vi "Lab Panel V4.82.vi"() -> ()   [LabVIEW 2013] (continued)
                n968 = Less?(x=w1637, y=2) -> (x < y?=w1640:bool)
                n969 = local read "DISP LAB02-2"() -> (w1642:T4)
                n970 = Unbundle(w1642) -> ("STATUS"=w1643:string)  [unwired: 2 out]
                n971 = Equal?(x=w1643, y="RUN") -> (x = y?=w1639:bool)
                n972 = And(x=w1639, y=w1640) -> (x .and. y?=w1638:bool)
                n973 = case shown="True" w1638 {
                  tunnel: w1642 -> [_ w1648]
                  tunnel: w1637 -> [_ w1652]
                  frame False {
                  }
                  frame True {
                    n974 = local read "SET LAB02-2"() -> (w1654:T5)
                    n975 = local read "TDMS LAB02-2"() -> (w1647:refnum<k34>)
                    n976 = Unbundle(w1648) -> ("CYCLE"=w1653:dbl)  [unwired: 2 out]
                    n977 = Unbundle(w1654) -> ("CYCLES"=w1645:dbl, "T-RISE mins"=w1651:dbl)  [unwired: 3 out]
                    n978 = case shown="\"T-RISE TEST\"" w1652 {
                      tunnel: w1651 -> [_ _ w1661]
                      tunnel: [w1656 w1658 w1661] -> w1650
                      tunnel: w1645 -> [w1656 w1658 _]
                      tunnel: ["CHART PASS" "CYCLE PASS" "T-RISE PASS"] -> w1649
                      frame "CHART TEST", Default {
                      }
                      frame "CYCLE TEST" {
                      }
                      frame "T-RISE TEST" {
                      }
                    }
                    n979 = Increment(x=w1645) -> (x+1=w1646:dbl)
                    n980 = Greater Or Equal?(x=w1653, y=w1646) -> (x >= y?=w1655:bool)
                    n981 = case shown="True" w1655 {
                      tunnel: w1650 -> [w1665 _]
                      tunnel: w1649 -> [w1664 _]
                      tunnel: w1648 -> [w1663 _]
                      tunnel: w1647 -> [w1662 _]
                      frame True {
                        n982 = stacked-sequence {
                          tunnel: w1665 -> [w1669 _]
                          tunnel: w1664 -> [w1667 w1673]
                          tunnel: w1663 -> [_ w1676]
                          tunnel: w1662 -> [w1666 _]
                          frame #0 {
                            n983 = Build Array(w1667) -> (w1670:string[])
                            n984 = Build Array(w1669) -> (w1668:dbl[])
                            n985 = TDMS Write(0:w1666, 5:"TEST PASS", 7:w1670, 9:w1668) -> (15:w1672:errorcluster)  [unwired: 2 in, 3 out]
                            n986 = local write "data file error"(w1672) -> ()
                          }
                          frame #1 {
                            n987 = Bundle(cluster=w1676, "STATUS"=w1673) -> (w1674:T4)  [unwired: 2 in]
                            n988 = local write "RESULT LAB02-2"(TRUE) -> ()
                            n989 = local write "DISP LAB02-2"(w1674) -> ()
                          }
                        }
                      }
                      frame False {
                      }
                    }
                  }
                }
              }
              frame #4 {
                # "LAB03-1"
                n990 = Less?(x=w1677, y=2) -> (x < y?=w1680:bool)
                n991 = local read "DISP LAB03-1"() -> (w1682:T4)
                n992 = Unbundle(w1682) -> ("STATUS"=w1683:string)  [unwired: 2 out]
                n993 = Equal?(x=w1683, y="RUN") -> (x = y?=w1679:bool)
                n994 = And(x=w1679, y=w1680) -> (x .and. y?=w1678:bool)
                n995 = case shown="True" w1678 {
                  tunnel: w1682 -> [_ w1688]
                  tunnel: w1677 -> [_ w1692]
                  frame False {
                  }
                  frame True {
                    n996 = local read "SET LAB03-1"() -> (w1694:T5)
                    n997 = local read "TDMS LAB03-1"() -> (w1687:refnum<k34>)
                    n998 = Unbundle(w1688) -> ("CYCLE"=w1693:dbl)  [unwired: 2 out]
                    n999 = Unbundle(w1694) -> ("CYCLES"=w1685:dbl, "T-RISE mins"=w1691:dbl)  [unwired: 3 out]
                    n1000 = case shown="\"T-RISE TEST\"" w1692 {
                      tunnel: w1691 -> [_ _ w1701]
                      tunnel: [w1696 w1698 w1701] -> w1690
                      tunnel: w1685 -> [w1696 w1698 _]
                      tunnel: ["CHART PASS" "CYCLE PASS" "T-RISE PASS"] -> w1689
                      frame "CHART TEST", Default {
                      }
                      frame "CYCLE TEST" {
                      }
                      frame "T-RISE TEST" {
                      }
                    }
                    n1001 = Increment(x=w1685) -> (x+1=w1686:dbl)
                    n1002 = Greater Or Equal?(x=w1693, y=w1686) -> (x >= y?=w1695:bool)
                    n1003 = case shown="True" w1695 {
                      tunnel: w1690 -> [w1705 _]
                      tunnel: w1689 -> [w1704 _]
                      tunnel: w1688 -> [w1703 _]
                      tunnel: w1687 -> [w1702 _]
                      frame True {
                        n1004 = stacked-sequence {
                          tunnel: w1705 -> [w1709 _]
                          tunnel: w1704 -> [w1707 w1713]
                          tunnel: w1703 -> [_ w1716]
                          tunnel: w1702 -> [w1706 _]
                          frame #0 {
                            n1005 = Build Array(w1707) -> (w1710:string[])
                            n1006 = Build Array(w1709) -> (w1708:dbl[])
                            n1007 = TDMS Write(0:w1706, 5:"TEST PASS", 7:w1710, 9:w1708) -> (15:w1712:errorcluster)  [unwired: 2 in, 3 out]
                            n1008 = local write "data file error"(w1712) -> ()
                          }
                          frame #1 {
                            n1009 = Bundle(cluster=w1716, "STATUS"=w1713) -> (w1714:T4)  [unwired: 2 in]
                            n1010 = local write "RESULT LAB03-1"(TRUE) -> ()
                            n1011 = local write "DISP LAB03-1"(w1714) -> ()
                          }
                        }
                      }
                      frame False {
                      }
                    }
                  }
                }
              }
              frame #5 {
                # "LAB03-2"
                n1012 = Less?(x=w1717, y=2) -> (x < y?=w1720:bool)
                n1013 = local read "DISP LAB03-2"() -> (w1722:T4)
                n1014 = Unbundle(w1722) -> ("STATUS"=w1723:string)  [unwired: 2 out]
                n1015 = Equal?(x=w1723, y="RUN") -> (x = y?=w1719:bool)
                n1016 = And(x=w1719, y=w1720) -> (x .and. y?=w1718:bool)
                n1017 = case shown="True" w1718 {
                  tunnel: w1722 -> [_ w1728]
                  tunnel: w1717 -> [_ w1732]
                  frame False {
                  }
                  frame True {
                    n1018 = local read "SET LAB03-2"() -> (w1734:T5)
                    n1019 = local read "TDMS LAB03-2"() -> (w1727:refnum<k34>)
                    n1020 = Unbundle(w1728) -> ("CYCLE"=w1733:dbl)  [unwired: 2 out]
                    n1021 = Unbundle(w1734) -> ("CYCLES"=w1725:dbl, "T-RISE mins"=w1731:dbl)  [unwired: 3 out]
                    n1022 = case shown="\"T-RISE TEST\"" w1732 {
                      tunnel: w1731 -> [_ _ w1741]
                      tunnel: [w1736 w1738 w1741] -> w1730
                      tunnel: w1725 -> [w1736 w1738 _]
                      tunnel: ["CHART PASS" "CYCLE PASS" "T-RISE PASS"] -> w1729
                      frame "CHART TEST", Default {
                      }
                      frame "CYCLE TEST" {
                      }
                      frame "T-RISE TEST" {
                      }
                    }
                    n1023 = Increment(x=w1725) -> (x+1=w1726:dbl)
                    n1024 = Greater Or Equal?(x=w1733, y=w1726) -> (x >= y?=w1735:bool)
                    n1025 = case shown="True" w1735 {
                      tunnel: w1730 -> [w1745 _]
                      tunnel: w1729 -> [w1744 _]
                      tunnel: w1728 -> [w1743 _]
                      tunnel: w1727 -> [w1742 _]
                      frame True {
                        n1026 = stacked-sequence {
                          tunnel: w1745 -> [w1749 _]
                          tunnel: w1744 -> [w1747 w1753]
                          tunnel: w1743 -> [_ w1756]
                          tunnel: w1742 -> [w1746 _]
                          frame #0 {
                            n1027 = Build Array(w1747) -> (w1750:string[])
                            n1028 = Build Array(w1749) -> (w1748:dbl[])
                            n1029 = TDMS Write(0:w1746, 5:"TEST PASS", 7:w1750, 9:w1748) -> (15:w1752:errorcluster)  [unwired: 2 in, 3 out]
                            n1030 = local write "data file error"(w1752) -> ()
                          }
                          frame #1 {
                            n1031 = Bundle(cluster=w1756, "STATUS"=w1753) -> (w1754:T4)  [unwired: 2 in]
                            n1032 = local write "RESULT LAB03-2"(TRUE) -> ()
                            n1033 = local write "DISP LAB03-2"(w1754) -> ()
                          }
                        }
                      }
                      frame False {
                      }
                    }
                  }
                }
              }
              frame #6 {
                # "LAB04-1"
                n1034 = Less?(x=w1757, y=2) -> (x < y?=w1760:bool)
                n1035 = local read "DISP LAB04-1"() -> (w1762:T4)
                n1036 = Unbundle(w1762) -> ("STATUS"=w1763:string)  [unwired: 2 out]
                n1037 = Equal?(x=w1763, y="RUN") -> (x = y?=w1759:bool)
                n1038 = And(x=w1759, y=w1760) -> (x .and. y?=w1758:bool)
                n1039 = case shown="True" w1758 {
                  tunnel: w1762 -> [_ w1768]
                  tunnel: w1757 -> [_ w1772]
                  frame False {
                  }
                  frame True {
                    n1040 = local read "SET LAB04-1"() -> (w1774:T5)
                    n1041 = local read "TDMS LAB04-1"() -> (w1767:refnum<k34>)
                    n1042 = Unbundle(w1768) -> ("CYCLE"=w1773:dbl)  [unwired: 2 out]
                    n1043 = Unbundle(w1774) -> ("CYCLES"=w1765:dbl, "T-RISE mins"=w1771:dbl)  [unwired: 3 out]
                    n1044 = case shown="\"T-RISE TEST\"" w1772 {
                      tunnel: w1771 -> [_ _ w1781]
                      tunnel: [w1776 w1778 w1781] -> w1770
                      tunnel: w1765 -> [w1776 w1778 _]
                      tunnel: ["CHART PASS" "CYCLE PASS" "T-RISE PASS"] -> w1769
                      frame "CHART TEST", Default {
                      }
                      frame "CYCLE TEST" {
                      }
                      frame "T-RISE TEST" {
                      }
                    }
                    n1045 = Increment(x=w1765) -> (x+1=w1766:dbl)
                    n1046 = Greater Or Equal?(x=w1773, y=w1766) -> (x >= y?=w1775:bool)
                    n1047 = case shown="True" w1775 {
                      tunnel: w1770 -> [w1785 _]
                      tunnel: w1769 -> [w1784 _]
                      tunnel: w1768 -> [w1783 _]
                      tunnel: w1767 -> [w1782 _]
                      frame True {
                        n1048 = stacked-sequence {
                          tunnel: w1785 -> [w1789 _]
                          tunnel: w1784 -> [w1787 w1793]
                          tunnel: w1783 -> [_ w1796]
                          tunnel: w1782 -> [w1786 _]
                          frame #0 {
                            n1049 = Build Array(w1787) -> (w1790:string[])
                            n1050 = Build Array(w1789) -> (w1788:dbl[])
                            n1051 = TDMS Write(0:w1786, 5:"TEST PASS", 7:w1790, 9:w1788) -> (15:w1792:errorcluster)  [unwired: 2 in, 3 out]
                            n1052 = local write "data file error"(w1792) -> ()
                          }
                          frame #1 {
                            n1053 = Bundle(cluster=w1796, "STATUS"=w1793) -> (w1794:T4)  [unwired: 2 in]
                            n1054 = local write "RESULT LAB04-1"(TRUE) -> ()
                            n1055 = local write "DISP LAB04-1"(w1794) -> ()
                          }
                        }
                      }
                      frame False {
                      }
                    }
                  }
                }
              }
              frame #7 {
                # "LAB04-2"
                n1056 = Less?(x=w1797, y=2) -> (x < y?=w1800:bool)
                n1057 = local read "DISP LAB04-2"() -> (w1802:T4)
                n1058 = Unbundle(w1802) -> ("STATUS"=w1803:string)  [unwired: 2 out]
                n1059 = Equal?(x=w1803, y="RUN") -> (x = y?=w1799:bool)
                n1060 = And(x=w1799, y=w1800) -> (x .and. y?=w1798:bool)
                n1061 = case shown="True" w1798 {
                  tunnel: w1802 -> [_ w1808]
                  tunnel: w1797 -> [_ w1812]
                  frame False {
                  }
                  frame True {
                    n1062 = local read "SET LAB04-2"() -> (w1814:T5)
                    n1063 = local read "TDMS LAB04-2"() -> (w1807:refnum<k34>)
                    n1064 = Unbundle(w1808) -> ("CYCLE"=w1813:dbl)  [unwired: 2 out]
                    n1065 = Unbundle(w1814) -> ("CYCLES"=w1805:dbl, "T-RISE mins"=w1811:dbl)  [unwired: 3 out]
                    n1066 = case shown="\"T-RISE TEST\"" w1812 {
                      tunnel: w1811 -> [_ _ w1821]
                      tunnel: [w1816 w1818 w1821] -> w1810
                      tunnel: w1805 -> [w1816 w1818 _]
                      tunnel: ["CHART PASS" "CYCLE PASS" "T-RISE PASS"] -> w1809
                      frame "CHART TEST", Default {
                      }
                      frame "CYCLE TEST" {
                      }
                      frame "T-RISE TEST" {
                      }
                    }
                    n1067 = Increment(x=w1805) -> (x+1=w1806:dbl)
                    n1068 = Greater Or Equal?(x=w1813, y=w1806) -> (x >= y?=w1815:bool)
                    n1069 = case shown="True" w1815 {
                      tunnel: w1810 -> [w1825 _]
                      tunnel: w1809 -> [w1824 _]
                      tunnel: w1808 -> [w1823 _]
                      tunnel: w1807 -> [w1822 _]
                      frame True {
                        n1070 = stacked-sequence {
                          tunnel: w1825 -> [w1829 _]
                          tunnel: w1824 -> [w1827 w1833]
                          tunnel: w1823 -> [_ w1836]
                          tunnel: w1822 -> [w1826 _]
                          frame #0 {
                            n1071 = Build Array(w1827) -> (w1830:string[])
                            n1072 = Build Array(w1829) -> (w1828:dbl[])
                            n1073 = TDMS Write(0:w1826, 5:"TEST PASS", 7:w1830, 9:w1828) -> (15:w1832:errorcluster)  [unwired: 2 in, 3 out]
                            n1074 = local write "data file error"(w1832) -> ()
                          }
                          frame #1 {
                            n1075 = Bundle(cluster=w1836, "STATUS"=w1833) -> (w1834:T4)  [unwired: 2 in]
                            n1076 = local write "RESULT LAB04-2"(TRUE) -> ()
                            n1077 = local write "DISP LAB04-2"(w1834) -> ()
                          }
                        }
                      }
                      frame False {
                      }
                    }
                  }
                }
              }
              frame #8 {
                # "LAB05-1"
                n1078 = Less?(x=w1837, y=2) -> (x < y?=w1840:bool)
                n1079 = local read "DISP LAB05-1"() -> (w1842:T4)
                n1080 = Unbundle(w1842) -> ("STATUS"=w1843:string)  [unwired: 2 out]
                n1081 = Equal?(x=w1843, y="RUN") -> (x = y?=w1839:bool)
                n1082 = And(x=w1839, y=w1840) -> (x .and. y?=w1838:bool)
                n1083 = case shown="True" w1838 {
                  tunnel: w1842 -> [_ w1848]
                  tunnel: w1837 -> [_ w1852]
                  frame False {
                  }
                  frame True {
                    n1084 = local read "SET LAB05-1"() -> (w1854:T5)
                    n1085 = local read "TDMS LAB05-1"() -> (w1847:refnum<k34>)
                    n1086 = Unbundle(w1848) -> ("CYCLE"=w1853:dbl)  [unwired: 2 out]
                    n1087 = Unbundle(w1854) -> ("CYCLES"=w1845:dbl, "T-RISE mins"=w1851:dbl)  [unwired: 3 out]
                    n1088 = case shown="\"T-RISE TEST\"" w1852 {
                      tunnel: w1851 -> [_ _ w1861]
                      tunnel: [w1856 w1858 w1861] -> w1850
                      tunnel: w1845 -> [w1856 w1858 _]
                      tunnel: ["CHART PASS" "CYCLE PASS" "T-RISE PASS"] -> w1849
                      frame "CHART TEST", Default {
                      }
                      frame "CYCLE TEST" {
                      }
                      frame "T-RISE TEST" {
                      }
                    }
                    n1089 = Increment(x=w1845) -> (x+1=w1846:dbl)
                    n1090 = Greater Or Equal?(x=w1853, y=w1846) -> (x >= y?=w1855:bool)
                    n1091 = case shown="True" w1855 {
                      tunnel: w1850 -> [w1865 _]
                      tunnel: w1849 -> [w1864 _]
                      tunnel: w1848 -> [w1863 _]
                      tunnel: w1847 -> [w1862 _]
                      frame True {
                        n1092 = stacked-sequence {
                          tunnel: w1865 -> [w1869 _]
                          tunnel: w1864 -> [w1867 w1873]
                          tunnel: w1863 -> [_ w1876]
                          tunnel: w1862 -> [w1866 _]
                          frame #0 {
                            n1093 = Build Array(w1867) -> (w1870:string[])
                            n1094 = Build Array(w1869) -> (w1868:dbl[])
                            n1095 = TDMS Write(0:w1866, 5:"TEST PASS", 7:w1870, 9:w1868) -> (15:w1872:errorcluster)  [unwired: 2 in, 3 out]
                            n1096 = local write "data file error"(w1872) -> ()
                          }
                          frame #1 {
                            n1097 = Bundle(cluster=w1876, "STATUS"=w1873) -> (w1874:T4)  [unwired: 2 in]
                            n1098 = local write "RESULT LAB05-1"(TRUE) -> ()
                            n1099 = local write "DISP LAB05-1"(w1874) -> ()
                          }
                        }
                      }
                      frame False {
                      }
                    }
                  }
                }
              }
              frame #9 {
                # "LAB05-2"
                n1100 = Less?(x=w1877, y=2) -> (x < y?=w1880:bool)
                n1101 = local read "DISP LAB05-2"() -> (w1882:T4)
                n1102 = Unbundle(w1882) -> ("STATUS"=w1883:string)  [unwired: 2 out]
                n1103 = Equal?(x=w1883, y="RUN") -> (x = y?=w1879:bool)
                n1104 = And(x=w1879, y=w1880) -> (x .and. y?=w1878:bool)
                n1105 = case shown="True" w1878 {
                  tunnel: w1882 -> [_ w1888]
                  tunnel: w1877 -> [_ w1892]
                  frame False {
                  }
                  frame True {
                    n1106 = local read "SET LAB05-2"() -> (w1894:T5)
                    n1107 = local read "TDMS LAB05-2"() -> (w1887:refnum<k34>)
                    n1108 = Unbundle(w1888) -> ("CYCLE"=w1893:dbl)  [unwired: 2 out]
                    n1109 = Unbundle(w1894) -> ("CYCLES"=w1885:dbl, "T-RISE mins"=w1891:dbl)  [unwired: 3 out]
                    n1110 = case shown="\"T-RISE TEST\"" w1892 {
                      tunnel: w1891 -> [_ _ w1901]
                      tunnel: [w1896 w1898 w1901] -> w1890
                      tunnel: w1885 -> [w1896 w1898 _]
                      tunnel: ["CHART PASS" "CYCLE PASS" "T-RISE PASS"] -> w1889
                      frame "CHART TEST", Default {
                      }
                      frame "CYCLE TEST" {
                      }
                      frame "T-RISE TEST" {
                      }
                    }
                    n1111 = Increment(x=w1885) -> (x+1=w1886:dbl)
                    n1112 = Greater Or Equal?(x=w1893, y=w1886) -> (x >= y?=w1895:bool)
                    n1113 = case shown="True" w1895 {
                      tunnel: w1890 -> [w1905 _]
                      tunnel: w1889 -> [w1904 _]
                      tunnel: w1888 -> [w1903 _]
                      tunnel: w1887 -> [w1902 _]
                      frame True {
                        n1114 = stacked-sequence {
                          tunnel: w1905 -> [w1909 _]
                          tunnel: w1904 -> [w1907 w1913]
                          tunnel: w1903 -> [_ w1916]
                          tunnel: w1902 -> [w1906 _]
                          frame #0 {
                            n1115 = Build Array(w1907) -> (w1910:string[])
                            n1116 = Build Array(w1909) -> (w1908:dbl[])
                            n1117 = TDMS Write(0:w1906, 5:"TEST PASS", 7:w1910, 9:w1908) -> (15:w1912:errorcluster)  [unwired: 2 in, 3 out]
                            n1118 = local write "data file error"(w1912) -> ()
                          }
                          frame #1 {
                            n1119 = Bundle(cluster=w1916, "STATUS"=w1913) -> (w1914:T4)  [unwired: 2 in]
                            n1120 = local write "RESULT LAB05-2"(TRUE) -> ()
                            n1121 = local write "DISP LAB05-2"(w1914) -> ()
                          }
                        }
                      }
                      frame False {
                      }
                    }
                  }
                }
              }
            }
          }
          frame #5 {
            # "check if test cycles reached for temperature rise test"
            n1122 = stacked-sequence {
              tunnel: w1946 -> [_ _ _ _ _ _ _ _ _ _]
              tunnel: w1945 -> [_ _ _ _ _ _ _ _ _ _]
              tunnel: w1944 -> [_ _ _ _ _ _ _ _ _ _]
              tunnel: w1943 -> [_ _ _ _ _ _ _ _ _ _]
              tunnel: w1942 -> [_ _ _ _ _ _ _ _ _ _]
              tunnel: w1941 -> [_ _ _ _ _ _ _ _ _ _]
              tunnel: w1940 -> [_ _ _ _ _ _ _ _ _ _]
              tunnel: w1939 -> [_ _ _ _ _ _ _ _ _ _]
              tunnel: w1938 -> [_ _ _ _ _ _ _ _ _ _]
              tunnel: w1937 -> [_ _ _ _ _ _ _ _ _ _]
              tunnel: w1936 -> [w1952 _ _ _ _ _ _ _ _ _]
              tunnel: w1926 -> [w1947 _ _ _ _ _ _ _ _ _]
              tunnel: w1935 -> [_ w1978 _ _ _ _ _ _ _ _]
              tunnel: w1934 -> [_ _ w2008 _ _ _ _ _ _ _]
              tunnel: w1933 -> [_ _ _ w2038 _ _ _ _ _ _]
              tunnel: w1932 -> [_ _ _ _ w2068 _ _ _ _ _]
              tunnel: w1931 -> [_ _ _ _ _ w2098 _ _ _ _]
              tunnel: w1930 -> [_ _ _ _ _ _ w2128 _ _ _]
              tunnel: w1929 -> [_ _ _ _ _ _ _ w2158 _ _]
              tunnel: w1928 -> [_ _ _ _ _ _ _ _ w2188 _]
              tunnel: w1927 -> [_ _ _ _ _ _ _ _ _ w2218]
              tunnel: w1925 -> [_ w1977 _ _ _ _ _ _ _ _]
              tunnel: w1924 -> [_ _ w2007 _ _ _ _ _ _ _]
              tunnel: w1923 -> [_ _ _ w2037 _ _ _ _ _ _]
              tunnel: w1922 -> [_ _ _ _ w2067 _ _ _ _ _]
              tunnel: w1921 -> [_ _ _ _ _ w2097 _ _ _ _]
              tunnel: w1920 -> [_ _ _ _ _ _ w2127 _ _ _]
              tunnel: w1919 -> [_ _ _ _ _ _ _ w2157 _ _]
              tunnel: w1918 -> [_ _ _ _ _ _ _ _ w2187 _]
              tunnel: w1917 -> [_ _ _ _ _ _ _ _ _ w2217]
              frame #0 {
                # "LAB01-1"
                n1123 = Equal?(x=w1952, y=2) -> (x = y?=w1950:bool)
                n1124 = local read "DISP LAB01-1"() -> (w1953:T4)
                n1125 = Unbundle(w1953) -> ("STATUS"=w1954:string)  [unwired: 2 out]
                n1126 = Equal?(x=w1954, y="RUN") -> (x = y?=w1949:bool)
                n1127 = And(x=w1949, y=w1950) -> (x .and. y?=w1948:bool)
                n1128 = case shown="True" w1948 {
                  tunnel: w1953 -> [_ w1957]
                  tunnel: w1947 -> [_ w1960]
                  frame False {
                  }
                  frame True {
                    n1129 = local read "SET LAB01-1"() -> (w1959:T5)
                    n1130 = local read "TDMS LAB01-1"() -> (w1956:refnum<k34>)
                    n1131 = Unbundle(w1957) -> ("CYCLE"=w1961:dbl)  [unwired: 2 out]
                    n1132 = Unbundle(w1959) -> ("T-RISE mins"=w1958:dbl)  [unwired: 4 out]
                    n1133 = Greater Or Equal?(x=w1961, y=w1960) -> (x >= y?=w1962:bool)
                    n1134 = case shown="True" w1962 {
                      tunnel: w1958 -> [w1965 _]
                      tunnel: w1957 -> [w1964 _]
                      tunnel: w1956 -> [w1963 _]
                      frame True {
                        n1135 = stacked-sequence {
                          tunnel: w1965 -> [w1968 _]
                          tunnel: w1964 -> [_ w1973]
                          tunnel: w1963 -> [w1966 _]
                          frame #0 {
                            n1136 = Build Array("T-RISE") -> (w1970:string[])
                            n1137 = Build Array(w1968) -> (w1969:dbl[])
                            n1138 = TDMS Write(0:w1966, 5:"TEST PASS", 7:w1970, 9:w1969) -> (15:w1972:errorcluster)  [unwired: 2 in, 3 out]
                            n1139 = local write "data file error"(w1972) -> ()
                          }
                          frame #1 {
                            n1140 = Bundle(cluster=w1973, "STATUS"="T-RISE PASS") -> (w1975:T4)  [unwired: 2 in]
                            n1141 = local write "RESULT LAB01-1"(TRUE) -> ()
                            n1142 = local write "DISP LAB01-1"(w1975) -> ()
                          }
                        }
                      }
                      frame False {
                      }
                    }
                  }
                }
              }
              frame #1 {
                # "LAB01-2"
                n1143 = Equal?(x=w1978, y=2) -> (x = y?=w1981:bool)
                n1144 = local read "DISP LAB01-2"() -> (w1983:T4)
                n1145 = Unbundle(w1983) -> ("STATUS"=w1984:string)  [unwired: 2 out]
                n1146 = Equal?(x=w1984, y="RUN") -> (x = y?=w1980:bool)
                n1147 = And(x=w1980, y=w1981) -> (x .and. y?=w1979:bool)
                n1148 = case shown="True" w1979 {
                  tunnel: w1983 -> [_ w1987]
                  tunnel: w1977 -> [_ w1990]
                  frame False {
                  }
                  frame True {
                    n1149 = local read "SET LAB01-2"() -> (w1989:T5)
                    n1150 = local read "TDMS LAB01-2"() -> (w1986:refnum<k34>)
                    n1151 = Unbundle(w1987) -> ("CYCLE"=w1991:dbl)  [unwired: 2 out]
                    n1152 = Unbundle(w1989) -> ("T-RISE mins"=w1988:dbl)  [unwired: 4 out]
                    n1153 = Greater Or Equal?(x=w1991, y=w1990) -> (x >= y?=w1992:bool)
                    n1154 = case shown="True" w1992 {
                      tunnel: w1988 -> [w1995 _]
                      tunnel: w1987 -> [w1994 _]
                      tunnel: w1986 -> [w1993 _]
                      frame True {
                        n1155 = stacked-sequence {
                          tunnel: w1995 -> [w1998 _]
                          tunnel: w1994 -> [_ w2003]
                          tunnel: w1993 -> [w1996 _]
                          frame #0 {
                            n1156 = Build Array("T-RISE") -> (w2000:string[])
                            n1157 = Build Array(w1998) -> (w1999:dbl[])
                            n1158 = TDMS Write(0:w1996, 5:"TEST PASS", 7:w2000, 9:w1999) -> (15:w2002:errorcluster)  [unwired: 2 in, 3 out]
                            n1159 = local write "data file error"(w2002) -> ()
                          }
                          frame #1 {
                            n1160 = Bundle(cluster=w2003, "STATUS"="T-RISE PASS") -> (w2005:T4)  [unwired: 2 in]
                            n1161 = local write "RESULT LAB01-2"(TRUE) -> ()
                            n1162 = local write "DISP LAB01-2"(w2005) -> ()
                          }
                        }
                      }
                      frame False {
                      }
                    }
                  }
                }
              }
              frame #2 {
                # "LAB02-1"
                n1163 = Equal?(x=w2008, y=2) -> (x = y?=w2011:bool)
                n1164 = local read "DISP LAB02-1"() -> (w2013:T4)
                n1165 = Unbundle(w2013) -> ("STATUS"=w2014:string)  [unwired: 2 out]
                n1166 = Equal?(x=w2014, y="RUN") -> (x = y?=w2010:bool)
                n1167 = And(x=w2010, y=w2011) -> (x .and. y?=w2009:bool)
                n1168 = case shown="True" w2009 {
                  tunnel: w2013 -> [_ w2017]
                  tunnel: w2007 -> [_ w2020]
                  frame False {
                  }
                  frame True {
                    n1169 = local read "SET LAB02-1"() -> (w2019:T5)
                    n1170 = local read "TDMS LAB02-1"() -> (w2016:refnum<k34>)
                    n1171 = Unbundle(w2017) -> ("CYCLE"=w2021:dbl)  [unwired: 2 out]
                    n1172 = Unbundle(w2019) -> ("T-RISE mins"=w2018:dbl)  [unwired: 4 out]
                    n1173 = Greater Or Equal?(x=w2021, y=w2020) -> (x >= y?=w2022:bool)
                    n1174 = case shown="True" w2022 {
                      tunnel: w2018 -> [w2025 _]
                      tunnel: w2017 -> [w2024 _]
                      tunnel: w2016 -> [w2023 _]
                      frame True {
                        n1175 = stacked-sequence {
                          tunnel: w2025 -> [w2028 _]
                          tunnel: w2024 -> [_ w2033]
                          tunnel: w2023 -> [w2026 _]
                          frame #0 {
                            n1176 = Build Array("T-RISE") -> (w2030:string[])
                            n1177 = Build Array(w2028) -> (w2029:dbl[])
                            n1178 = TDMS Write(0:w2026, 5:"TEST PASS", 7:w2030, 9:w2029) -> (15:w2032:errorcluster)  [unwired: 2 in, 3 out]
                            n1179 = local write "data file error"(w2032) -> ()
                          }
                          frame #1 {
                            n1180 = Bundle(cluster=w2033, "STATUS"="T-RISE PASS") -> (w2035:T4)  [unwired: 2 in]
                            n1181 = local write "RESULT LAB02-1"(TRUE) -> ()
                            n1182 = local write "DISP LAB02-1"(w2035) -> ()
                          }
                        }
                      }
                      frame False {
                      }
                    }
                  }
                }
              }
              frame #3 {
                # "LAB02-2"
                n1183 = Equal?(x=w2038, y=2) -> (x = y?=w2041:bool)
                n1184 = local read "DISP LAB02-2"() -> (w2043:T4)
                n1185 = Unbundle(w2043) -> ("STATUS"=w2044:string)  [unwired: 2 out]
                n1186 = Equal?(x=w2044, y="RUN") -> (x = y?=w2040:bool)
                n1187 = And(x=w2040, y=w2041) -> (x .and. y?=w2039:bool)
                n1188 = case shown="True" w2039 {
                  tunnel: w2043 -> [_ w2047]
                  tunnel: w2037 -> [_ w2050]
                  frame False {
                  }
                  frame True {
                    n1189 = local read "SET LAB02-2"() -> (w2049:T5)
                    n1190 = local read "TDMS LAB02-2"() -> (w2046:refnum<k34>)
                    n1191 = Unbundle(w2047) -> ("CYCLE"=w2051:dbl)  [unwired: 2 out]
                    n1192 = Unbundle(w2049) -> ("T-RISE mins"=w2048:dbl)  [unwired: 4 out]
                    n1193 = Greater Or Equal?(x=w2051, y=w2050) -> (x >= y?=w2052:bool)
                    n1194 = case shown="True" w2052 {
                      tunnel: w2048 -> [w2055 _]
                      tunnel: w2047 -> [w2054 _]
                      tunnel: w2046 -> [w2053 _]
                      frame True {
                        n1195 = stacked-sequence {
                          tunnel: w2055 -> [w2058 _]
                          tunnel: w2054 -> [_ w2063]
                          tunnel: w2053 -> [w2056 _]
                          frame #0 {
                            n1196 = Build Array("T-RISE") -> (w2060:string[])
                            n1197 = Build Array(w2058) -> (w2059:dbl[])
                            n1198 = TDMS Write(0:w2056, 5:"TEST PASS", 7:w2060, 9:w2059) -> (15:w2062:errorcluster)  [unwired: 2 in, 3 out]
                            n1199 = local write "data file error"(w2062) -> ()
                          }
                          frame #1 {
                            n1200 = Bundle(cluster=w2063, "STATUS"="T-RISE PASS") -> (w2065:T4)  [unwired: 2 in]
                            n1201 = local write "RESULT LAB02-2"(TRUE) -> ()
                            n1202 = local write "DISP LAB02-2"(w2065) -> ()
                          }
                        }
                      }
                      frame False {
                      }
                    }
                  }
                }
              }
              frame #4 {
                # "LAB03-1"
                n1203 = Equal?(x=w2068, y=2) -> (x = y?=w2071:bool)
                n1204 = local read "DISP LAB03-1"() -> (w2073:T4)
                n1205 = Unbundle(w2073) -> ("STATUS"=w2074:string)  [unwired: 2 out]
                n1206 = Equal?(x=w2074, y="RUN") -> (x = y?=w2070:bool)
                n1207 = And(x=w2070, y=w2071) -> (x .and. y?=w2069:bool)
                n1208 = case shown="True" w2069 {
                  tunnel: w2073 -> [_ w2077]
                  tunnel: w2067 -> [_ w2080]
                  frame False {
                  }
                  frame True {
                    n1209 = local read "SET LAB03-1"() -> (w2079:T5)
                    n1210 = local read "TDMS LAB03-1"() -> (w2076:refnum<k34>)
                    n1211 = Unbundle(w2077) -> ("CYCLE"=w2081:dbl)  [unwired: 2 out]
                    n1212 = Unbundle(w2079) -> ("T-RISE mins"=w2078:dbl)  [unwired: 4 out]
                    n1213 = Greater Or Equal?(x=w2081, y=w2080) -> (x >= y?=w2082:bool)
                    n1214 = case shown="True" w2082 {
                      tunnel: w2078 -> [w2085 _]
                      tunnel: w2077 -> [w2084 _]
                      tunnel: w2076 -> [w2083 _]
                      frame True {
                        n1215 = stacked-sequence {
                          tunnel: w2085 -> [w2088 _]
                          tunnel: w2084 -> [_ w2093]
                          tunnel: w2083 -> [w2086 _]
                          frame #0 {
                            n1216 = Build Array("T-RISE") -> (w2090:string[])
                            n1217 = Build Array(w2088) -> (w2089:dbl[])
                            n1218 = TDMS Write(0:w2086, 5:"TEST PASS", 7:w2090, 9:w2089) -> (15:w2092:errorcluster)  [unwired: 2 in, 3 out]
                            n1219 = local write "data file error"(w2092) -> ()
                          }
                          frame #1 {
                            n1220 = Bundle(cluster=w2093, "STATUS"="T-RISE PASS") -> (w2095:T4)  [unwired: 2 in]
                            n1221 = local write "RESULT LAB03-1"(TRUE) -> ()
                            n1222 = local write "DISP LAB03-1"(w2095) -> ()
                          }
                        }
                      }
                      frame False {
                      }
                    }
                  }
                }
              }
              frame #5 {
                # "LAB03-2"
                n1223 = Equal?(x=w2098, y=2) -> (x = y?=w2101:bool)
                n1224 = local read "DISP LAB03-2"() -> (w2103:T4)
                n1225 = Unbundle(w2103) -> ("STATUS"=w2104:string)  [unwired: 2 out]
                n1226 = Equal?(x=w2104, y="RUN") -> (x = y?=w2100:bool)
                n1227 = And(x=w2100, y=w2101) -> (x .and. y?=w2099:bool)
                n1228 = case shown="True" w2099 {
                  tunnel: w2103 -> [_ w2107]
                  tunnel: w2097 -> [_ w2110]
                  frame False {
                  }
                  frame True {
                    n1229 = local read "SET LAB03-2"() -> (w2109:T5)
                    n1230 = local read "TDMS LAB03-2"() -> (w2106:refnum<k34>)
                    n1231 = Unbundle(w2107) -> ("CYCLE"=w2111:dbl)  [unwired: 2 out]
                    n1232 = Unbundle(w2109) -> ("T-RISE mins"=w2108:dbl)  [unwired: 4 out]
                    n1233 = Greater Or Equal?(x=w2111, y=w2110) -> (x >= y?=w2112:bool)
                    n1234 = case shown="True" w2112 {
                      tunnel: w2108 -> [w2115 _]
                      tunnel: w2107 -> [w2114 _]
                      tunnel: w2106 -> [w2113 _]
                      frame True {
                        n1235 = stacked-sequence {
                          tunnel: w2115 -> [w2118 _]
                          tunnel: w2114 -> [_ w2123]
                          tunnel: w2113 -> [w2116 _]
                          frame #0 {
                            n1236 = Build Array("T-RISE") -> (w2120:string[])
                            n1237 = Build Array(w2118) -> (w2119:dbl[])
                            n1238 = TDMS Write(0:w2116, 5:"TEST PASS", 7:w2120, 9:w2119) -> (15:w2122:errorcluster)  [unwired: 2 in, 3 out]
                            n1239 = local write "data file error"(w2122) -> ()
                          }
                          frame #1 {
                            n1240 = Bundle(cluster=w2123, "STATUS"="T-RISE PASS") -> (w2125:T4)  [unwired: 2 in]
                            n1241 = local write "RESULT LAB03-2"(TRUE) -> ()
                            n1242 = local write "DISP LAB03-2"(w2125) -> ()
                          }
                        }
                      }
                      frame False {
                      }
                    }
                  }
                }
              }
              frame #6 {
                # "LAB04-1"
                n1243 = Equal?(x=w2128, y=2) -> (x = y?=w2131:bool)
                n1244 = local read "DISP LAB04-1"() -> (w2133:T4)
                n1245 = Unbundle(w2133) -> ("STATUS"=w2134:string)  [unwired: 2 out]
                n1246 = Equal?(x=w2134, y="RUN") -> (x = y?=w2130:bool)
                n1247 = And(x=w2130, y=w2131) -> (x .and. y?=w2129:bool)
                n1248 = case shown="True" w2129 {
                  tunnel: w2133 -> [_ w2137]
                  tunnel: w2127 -> [_ w2140]
                  frame False {
                  }
                  frame True {
                    n1249 = local read "SET LAB04-1"() -> (w2139:T5)
                    n1250 = local read "TDMS LAB04-1"() -> (w2136:refnum<k34>)
                    n1251 = Unbundle(w2137) -> ("CYCLE"=w2141:dbl)  [unwired: 2 out]
                    n1252 = Unbundle(w2139) -> ("T-RISE mins"=w2138:dbl)  [unwired: 4 out]
                    n1253 = Greater Or Equal?(x=w2141, y=w2140) -> (x >= y?=w2142:bool)
                    n1254 = case shown="True" w2142 {
                      tunnel: w2138 -> [w2145 _]
                      tunnel: w2137 -> [w2144 _]
                      tunnel: w2136 -> [w2143 _]
                      frame True {
                        n1255 = stacked-sequence {
                          tunnel: w2145 -> [w2148 _]
                          tunnel: w2144 -> [_ w2153]
                          tunnel: w2143 -> [w2146 _]
                          frame #0 {
                            n1256 = Build Array("T-RISE") -> (w2150:string[])
                            n1257 = Build Array(w2148) -> (w2149:dbl[])
                            n1258 = TDMS Write(0:w2146, 5:"TEST PASS", 7:w2150, 9:w2149) -> (15:w2152:errorcluster)  [unwired: 2 in, 3 out]
                            n1259 = local write "data file error"(w2152) -> ()
                          }
                          frame #1 {
                            n1260 = Bundle(cluster=w2153, "STATUS"="T-RISE PASS") -> (w2155:T4)  [unwired: 2 in]
                            n1261 = local write "RESULT LAB04-1"(TRUE) -> ()
                            n1262 = local write "DISP LAB04-1"(w2155) -> ()
                          }
                        }
                      }
                      frame False {
                      }
                    }
                  }
                }
              }
              frame #7 {
                # "LAB04-2"
                n1263 = Equal?(x=w2158, y=2) -> (x = y?=w2161:bool)
                n1264 = local read "DISP LAB04-2"() -> (w2163:T4)
                n1265 = Unbundle(w2163) -> ("STATUS"=w2164:string)  [unwired: 2 out]
                n1266 = Equal?(x=w2164, y="RUN") -> (x = y?=w2160:bool)
                n1267 = And(x=w2160, y=w2161) -> (x .and. y?=w2159:bool)
                n1268 = case shown="True" w2159 {
                  tunnel: w2163 -> [_ w2167]
                  tunnel: w2157 -> [_ w2170]
                  frame False {
                  }
                  frame True {
                    n1269 = local read "SET LAB04-2"() -> (w2169:T5)
                    n1270 = local read "TDMS LAB04-2"() -> (w2166:refnum<k34>)
                    n1271 = Unbundle(w2167) -> ("CYCLE"=w2171:dbl)  [unwired: 2 out]
                    n1272 = Unbundle(w2169) -> ("T-RISE mins"=w2168:dbl)  [unwired: 4 out]
                    n1273 = Greater Or Equal?(x=w2171, y=w2170) -> (x >= y?=w2172:bool)
                    n1274 = case shown="True" w2172 {
                      tunnel: w2168 -> [w2175 _]
                      tunnel: w2167 -> [w2174 _]
                      tunnel: w2166 -> [w2173 _]
                      frame True {
                        n1275 = stacked-sequence {
                          tunnel: w2175 -> [w2178 _]
                          tunnel: w2174 -> [_ w2183]
                          tunnel: w2173 -> [w2176 _]
                          frame #0 {
                            n1276 = Build Array("T-RISE") -> (w2180:string[])
                            n1277 = Build Array(w2178) -> (w2179:dbl[])
                            n1278 = TDMS Write(0:w2176, 5:"TEST PASS", 7:w2180, 9:w2179) -> (15:w2182:errorcluster)  [unwired: 2 in, 3 out]
                            n1279 = local write "data file error"(w2182) -> ()
                          }
                          frame #1 {
                            n1280 = Bundle(cluster=w2183, "STATUS"="T-RISE PASS") -> (w2185:T4)  [unwired: 2 in]
                            n1281 = local write "RESULT LAB04-2"(TRUE) -> ()
                            n1282 = local write "DISP LAB04-2"(w2185) -> ()
                          }
                        }
                      }
                      frame False {
                      }
                    }
                  }
                }
              }
              frame #8 {
                # "LAB05-1"
                n1283 = Equal?(x=w2188, y=2) -> (x = y?=w2191:bool)
                n1284 = local read "DISP LAB05-1"() -> (w2193:T4)
                n1285 = Unbundle(w2193) -> ("STATUS"=w2194:string)  [unwired: 2 out]
                n1286 = Equal?(x=w2194, y="RUN") -> (x = y?=w2190:bool)
                n1287 = And(x=w2190, y=w2191) -> (x .and. y?=w2189:bool)
                n1288 = case shown="True" w2189 {
                  tunnel: w2193 -> [_ w2197]
                  tunnel: w2187 -> [_ w2200]
                  frame False {
                  }
                  frame True {
                    n1289 = local read "SET LAB05-1"() -> (w2199:T5)
                    n1290 = local read "TDMS LAB05-1"() -> (w2196:refnum<k34>)
                    n1291 = Unbundle(w2197) -> ("CYCLE"=w2201:dbl)  [unwired: 2 out]
                    n1292 = Unbundle(w2199) -> ("T-RISE mins"=w2198:dbl)  [unwired: 4 out]
                    n1293 = Greater Or Equal?(x=w2201, y=w2200) -> (x >= y?=w2202:bool)
                    n1294 = case shown="True" w2202 {
                      tunnel: w2198 -> [w2205 _]
                      tunnel: w2197 -> [w2204 _]
                      tunnel: w2196 -> [w2203 _]
                      frame True {
                        n1295 = stacked-sequence {
                          tunnel: w2205 -> [w2208 _]
                          tunnel: w2204 -> [_ w2213]
                          tunnel: w2203 -> [w2206 _]
                          frame #0 {
                            n1296 = Build Array("T-RISE") -> (w2210:string[])
                            n1297 = Build Array(w2208) -> (w2209:dbl[])
                            n1298 = TDMS Write(0:w2206, 5:"TEST PASS", 7:w2210, 9:w2209) -> (15:w2212:errorcluster)  [unwired: 2 in, 3 out]
                            n1299 = local write "data file error"(w2212) -> ()
                          }
                          frame #1 {
                            n1300 = Bundle(cluster=w2213, "STATUS"="T-RISE PASS") -> (w2215:T4)  [unwired: 2 in]
                            n1301 = local write "RESULT LAB05-1"(TRUE) -> ()
                            n1302 = local write "DISP LAB05-1"(w2215) -> ()
                          }
                        }
                      }
                      frame False {
                      }
                    }
                  }
                }
              }
              frame #9 {
                # "LAB05-2"
                n1303 = Equal?(x=w2218, y=2) -> (x = y?=w2221:bool)
                n1304 = local read "DISP LAB05-2"() -> (w2223:T4)
                n1305 = Unbundle(w2223) -> ("STATUS"=w2224:string)  [unwired: 2 out]
                n1306 = Equal?(x=w2224, y="RUN") -> (x = y?=w2220:bool)
                n1307 = And(x=w2220, y=w2221) -> (x .and. y?=w2219:bool)
                n1308 = case shown="True" w2219 {
                  tunnel: w2223 -> [_ w2227]
                  tunnel: w2217 -> [_ w2230]
                  frame False {
                  }
                  frame True {
                    n1309 = local read "SET LAB05-2"() -> (w2229:T5)
                    n1310 = local read "TDMS LAB05-2"() -> (w2226:refnum<k34>)
                    n1311 = Unbundle(w2227) -> ("CYCLE"=w2231:dbl)  [unwired: 2 out]
                    n1312 = Unbundle(w2229) -> ("T-RISE mins"=w2228:dbl)  [unwired: 4 out]
                    n1313 = Greater Or Equal?(x=w2231, y=w2230) -> (x >= y?=w2232:bool)
                    n1314 = case shown="True" w2232 {
                      tunnel: w2228 -> [w2235 _]
                      tunnel: w2227 -> [w2234 _]
                      tunnel: w2226 -> [w2233 _]
                      frame True {
                        n1315 = stacked-sequence {
                          tunnel: w2235 -> [w2238 _]
                          tunnel: w2234 -> [_ w2243]
                          tunnel: w2233 -> [w2236 _]
                          frame #0 {
                            n1316 = Build Array("T-RISE") -> (w2240:string[])
                            n1317 = Build Array(w2238) -> (w2239:dbl[])
                            n1318 = TDMS Write(0:w2236, 5:"TEST PASS", 7:w2240, 9:w2239) -> (15:w2242:errorcluster)  [unwired: 2 in, 3 out]
                            n1319 = local write "data file error"(w2242) -> ()
                          }
                          frame #1 {
                            n1320 = Bundle(cluster=w2243, "STATUS"="T-RISE PASS") -> (w2245:T4)  [unwired: 2 in]
                            n1321 = local write "RESULT LAB05-2"(TRUE) -> ()
                            n1322 = local write "DISP LAB05-2"(w2245) -> ()
                          }
                        }
                      }
                      frame False {
                      }
                    }
                  }
                }
              }
            }
          }
          frame #6 {
            # "end test & close test files"
            n1323 = stacked-sequence {
              tunnel: w2256 -> [_ _ _ _ _ _ _ _ _ _]
              tunnel: w2257 -> [_ _ _ _ _ _ _ _ _ _]
              tunnel: w2255 -> [_ _ _ _ _ _ _ _ _ _]
              tunnel: w2254 -> [_ _ _ _ _ _ _ _ _ _]
              tunnel: w2253 -> [_ _ _ _ _ _ _ _ _ _]
              tunnel: w2252 -> [_ _ _ _ _ _ _ _ _ _]
              tunnel: w2251 -> [_ _ _ _ _ _ _ _ _ _]
              tunnel: w2250 -> [_ _ _ _ _ _ _ _ _ _]
              tunnel: w2249 -> [_ _ _ _ _ _ _ _ _ _]
              tunnel: w2248 -> [_ _ _ _ _ _ _ _ _ _]
              frame #0 {
                # "LAB01-1"
                n1324 = local read "DISP LAB01-1"() -> (w2261:T4)
                n1325 = local read "run lab01-1"() -> (w2258:bool)
                n1326 = local read "TDMS LAB01-1"() -> (w2259:refnum<k34>)
                n1327 = Unbundle(w2261) -> ("CYCLE"=w2262:dbl, "STATUS"=w2260:string)  [unwired: 1 out]
                n1328 = case shown="True" w2258 {
                  tunnel: w2262 -> [_ w2266]
                  tunnel: w2261 -> [_ w2265]
                  tunnel: w2260 -> [_ w2264]
                  tunnel: w2259 -> [_ w2263]
                  frame False {
                  }
                  frame True {
                    n1329 = Not Equal?(x=w2264, y="RUN") -> (x != y?=w2267:bool)
                    n1330 = Greater?(x=w2266, y=2.0) -> (0:w2269:bool)
                    n1331 = And(x=w2269, y=w2267) -> (x .and. y?=w2268:bool)
                    n1332 = case shown="True" w2268 {
                      tunnel: w2265 -> [_ w2273]
                      tunnel: w2263 -> [_ w2272]
                      frame False {
                      }
                      frame True {
                        n1333 = stacked-sequence {
                          tunnel: w2273 -> [w2277 _ _]
                          tunnel: w2272 -> [_ w2279 _]
                          frame #0 {
                            w2274 = FALSE
                            n1334 = local write "mail control"("END") -> ()
